vi "Receive Boolean.vi"(8 "error in (no error)":errorcluster, 10 "Broadcast Boolean Msg":refnum<class "Broadcast Boolean Msg.lvclass">, 11 "IModel In":refnum<class "IModel.lvclass">) -> (0 "error out":errorcluster, 3 "IModel Out":refnum<class "IModel.lvclass">)   [LabVIEW 2015, in "IModel.lvlib" / "IModel.lvclass"]
uses:
  IModel.lvclass
  IViewable/IViewable Messages/Broadcast Boolean Msg/Broadcast Boolean Msg.lvclass
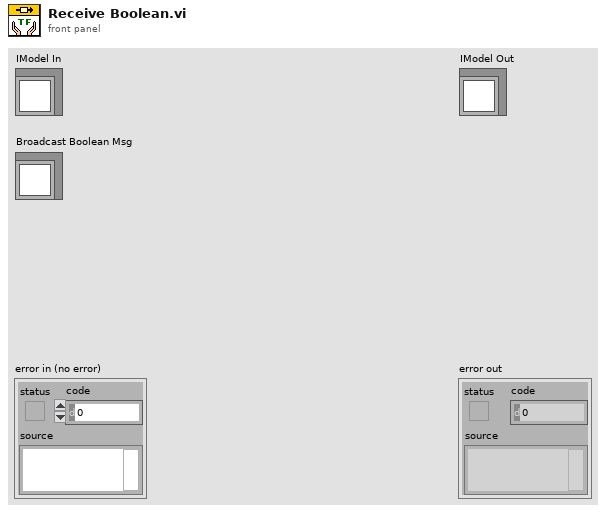
[diagram p1: front panel]
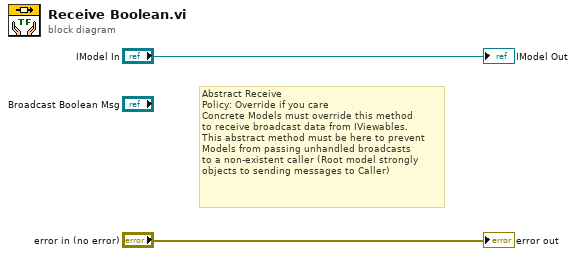
[diagram p0: block diagram]
diagram:
  # "Abstract Receive\nPolicy: Override if you care\nConcrete Models must override this method\nto receive broadcast data from IViewables.\nThis abstract method must be here to prevent\nModels from passing unhandled broadcasts\nto a non-existent caller (Root model strongly\nobjects to sending messages to Caller)"
  "error out" <- "error in (no error)"
  "IModel Out" <- "IModel In"
